vi "Request Termination.vi"(8 "error in (no error)":errorcluster, 10 "force kill":bool=TRUE, 11 "subprocess in":refnum<class "Subprocess.lvclass">) -> (0 "error out":errorcluster, 3 "subprocess out":refnum<class "Subprocess.lvclass">)   [LabVIEW 2020, in "NI_Subprocess.lvlib" / "Subprocess.lvclass"]
doc: "Signal a subprocess to exit. This happens asynchronously; use <b>Wait for exit.vi</b> to ensure the subprocess has exited. If <b>force kill?</b> is true, the subprocess is forcibly terminated."
uses:
  <vilib>/Subprocess/Subprocess/Subprocess.lvclass
  <vilib>/Subprocess/Subprocess/Subprocess.lvclass/Subprocess.ctl
  <vilib>/Utility/error.llb/Error Cluster From Error Code.vi
  <vilib>/ErrorRing/Error Ring.xnode
  lviosrg.dll
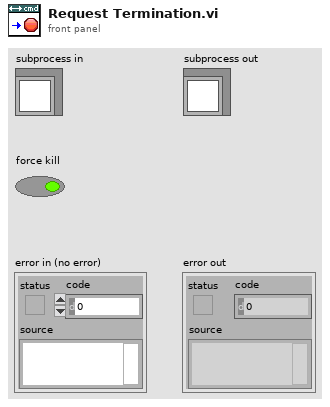
[diagram p1: front panel]
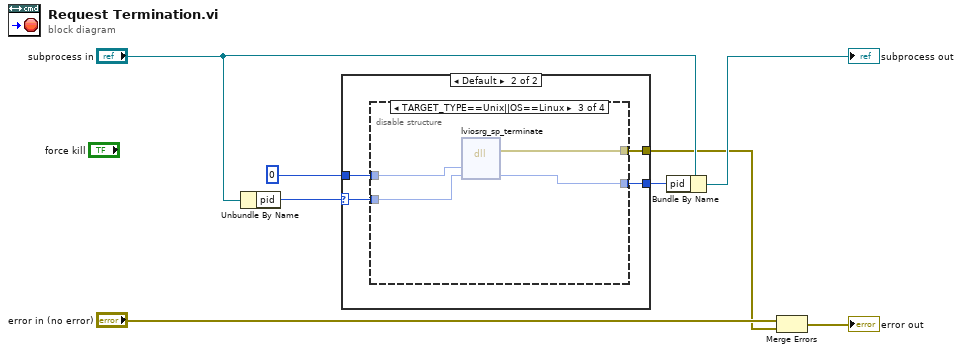
[diagram p0: block diagram]
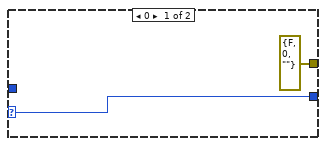
[diagram p2: hidden frame]
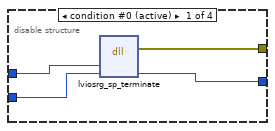
[diagram p3: hidden frame]
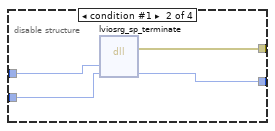
[diagram p4: hidden frame]
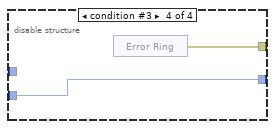
[diagram p5: hidden frame]
diagram:
  n1 = Unbundle By Name("subprocess in") -> ("pid"=w1:u64)
  n2 = case shown="Default" w1 {
    selector: w1 -> [w10 w11]
    tunnel: [w10 w14] -> w7
    tunnel: 0 ("errno") -> [_ w13]
    tunnel: [errorcluster {"status"=FALSE, "code"=0, "source"=""} ("error out") w12] -> w3
    frame 0 {
    }
    frame Default {
      n3 = disable-structure shown="TARGET_TYPE==Unix||OS==Linux" {
        disable-tunnel: w11 -> [w18 w22 w26 w28]
        disable-tunnel: [w17 w21 w25 w28] -> w14
        disable-tunnel: w13 -> [w16 w20 w24 _]
        disable-tunnel: [w15 w19 w23 w27] -> w12
        frame condition #0 (active) {
          n4 = dll-call lib="lviosrg.dll" fn="lviosrg_sp_terminate"("errno"=w16, "process"=w18) -> (error out=w15:errorcluster, "process"=w17:u64)  [unwired: 5 in, 1 out]
        }
        frame condition #1 {
          n5 = dll-call lib="lviosrg.*" fn="lviosrg_sp_terminate"("errno"=w20, "process"=w22) -> (error out=w19:errorcluster, "process"=w21:u64)  [unwired: 5 in, 1 out]
        }
        frame condition #2 {
          n6 = dll-call lib="lviosrg.*" fn="lviosrg_sp_terminate"("errno"=w24, "process"=w26) -> (error out=w23:errorcluster, "process"=w25:u64)  [unwired: 5 in, 1 out]
        }
        frame condition #3 {
          n7 = xnode "Error Ring"() -> ("error out"=w27:errorcluster)
        }
      }
    }
  }
  n8 = Bundle By Name(cluster="subprocess in", "pid"=w7) -> (→"subprocess out":refnum<class "Subprocess.lvclass">)
  n9 = Merge Errors("error in (no error)", w3) -> (→"error out":errorcluster)
